vi "test write new frame.vi"() -> ()   [LabVIEW 2018, in "Data Parser.lvclass"]
uses:
  Data Parser.lvclass
  frame data.ctl
  frame title.ctl
  frame basic data.ctl
  frame o data.ctl
  frame bp data.ctl
  frame c data.ctl
  frame w data.ctl
  frame i data.ctl
  frame b data.ctl
panel:
  in  "frame data":T1
  out "new":bool
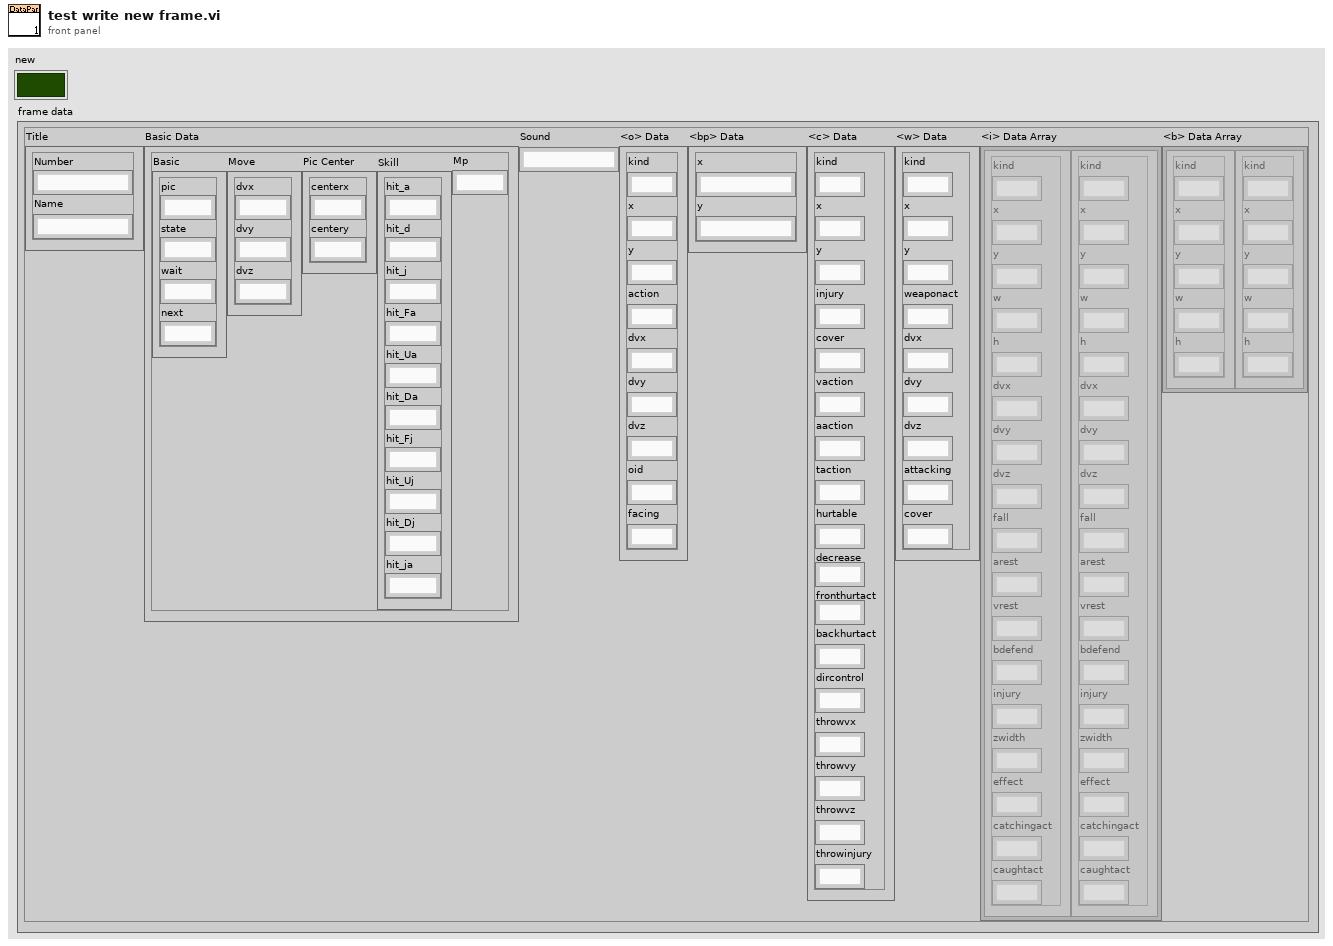
[diagram p1: front panel]
types:
  T1 = typedef "Data Parser.lvclass/frame data.ctl" = cluster{"Title":T2, "Basic Data":T3, "Sound":string, "<o> Data":T4, "<bp> Data":T5, "<c> Data":T6, "<w> Data":T7, "<i> Data Array":T8[], "<b> Data Array":T9[]}
  T2 = typedef "Data Parser.lvclass/frame title.ctl" = cluster{"Number":string, "Name":string}
  T3 = typedef "Data Parser.lvclass/frame basic data.ctl" = cluster{"Basic":cluster{"pic":string, "state":string, "wait":string, "next":string}, "Move":cluster{"dvx":string, "dvy":string, "dvz":string}, "Pic Center":cluster{"centerx":string, "centery":string}, "Skill":cluster{"hit_a":string, "hit_d":string, "hit_j":string, "hit_Fa":string, "hit_Ua":string, "hit_Da":string, "hit_Fj":string, "hit_Uj":string, "hit_Dj":string, "hit_ja":string}, "Mp":string}
  T4 = typedef "Data Parser.lvclass/frame o data.ctl" = cluster{"kind":string, "x":string, "y":string, "action":string, "dvx":string, "dvy":string, "dvz":string, "oid":string, "facing":string}
  T5 = typedef "Data Parser.lvclass/frame bp data.ctl" = cluster{"x":string, "y":string}
  T6 = typedef "Data Parser.lvclass/frame c data.ctl" = cluster{"kind":string, "x":string, "y":string, "injury":string, "cover":string, "vaction":string, "aaction":string, "taction":string, "hurtable":string, "decrease":string, "fronthurtact":string, "backhurtact":string, "dircontrol":string, "throwvx":string, "throwvy":string, "throwvz":string, "throwinjury":string}
  T7 = typedef "Data Parser.lvclass/frame w data.ctl" = cluster{"kind":string, "x":string, "y":string, "weaponact":string, "dvx":string, "dvy":string, "dvz":string, "attacking":string, "cover":string}
  T8 = typedef "Data Parser.lvclass/frame i data.ctl" = cluster{"kind":string, "x":string, "y":string, "w":string, "h":string, "dvx":string, "dvy":string, "dvz":string, "fall":string, "arest":string, "vrest":string, "bdefend":string, "injury":string, "zwidth":string, "effect":string, "catchingact":string, "caughtact":string}
  T9 = typedef "Data Parser.lvclass/frame b data.ctl" = cluster{"kind":string, "x":string, "y":string, "w":string, "h":string}
  T10 = enum16{"open", "replace", "create", "open or create", "replace or create", "replace or create with confirmation"}
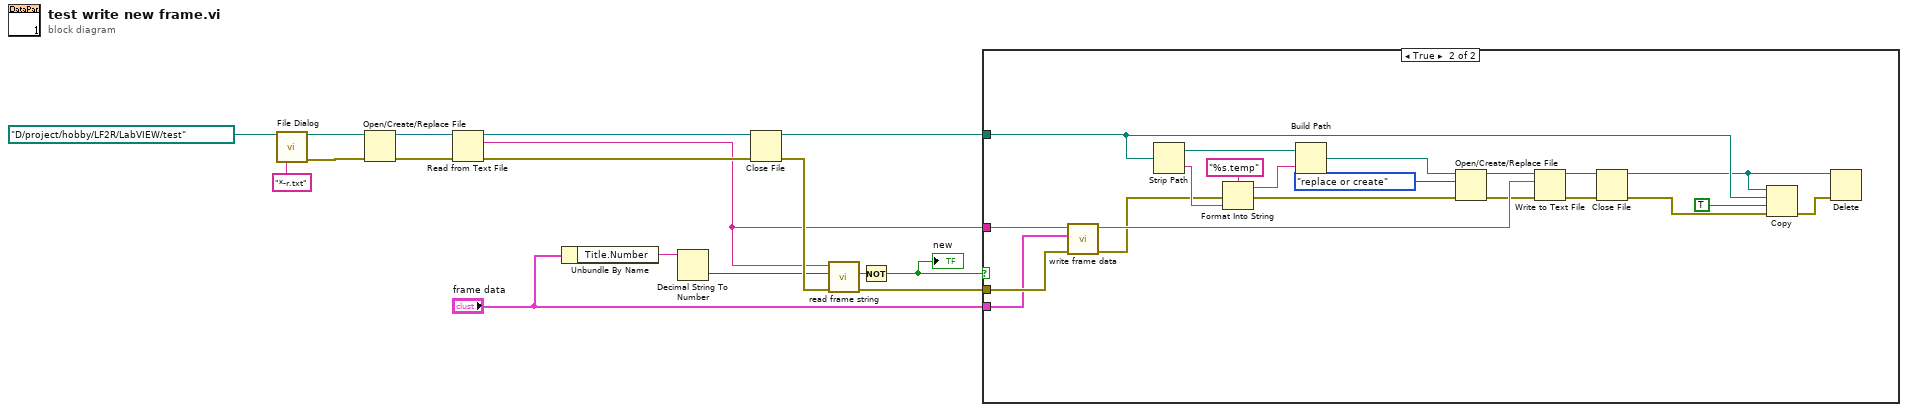
[diagram p0: block diagram]
diagram:
  n1 = call "File Dialog"("start path"=path "D:/project/hobby/LF2R/LabVIEW/test", "pattern (all files)"="*-r.txt") -> ("selected path"=w15:path, "error out"=w14:errorcluster)  [unwired: 10 in, 2 out]
  n2 = Open/Create/Replace File(file path (use dialog)=w15, error in=w14) -> (refnum out=w17:refnum<file>, error out=w16:errorcluster)  [unwired: 4 in, 1 out]
  n3 = Read from Text File(file (use dialog)=w17, error in=w16) -> (refnum out=w11:refnum<file>, text=w7:string, error out=w10:errorcluster)  [unwired: 2 in, 1 out]
  n4 = Unbundle By Name("frame data") -> ("Title.Number"=w2:string)
  n5 = Decimal String To Number(string=w2) -> (number=w1:i32)  [unwired: 2 in, 1 out]
  n6 = Close File(refnum=w11, error in=w10) -> (path=w8:path, error out=w9:errorcluster)
  n7 = call "read frame string.vi"("error in"=w9, "frame number"=w1, "file string"=w7) -> ("error out"=w4:errorcluster, "found"=w6:bool)  [unwired: 5 in, 2 out]
  n8 = Not(x=w6) -> (.not. x?=w5:bool)
  "new" <- w5
  n9 = case shown="True" w5 {
    tunnel: w8 -> [_ w38]
    tunnel: w7 -> [_ w37]
    tunnel: "frame data" -> [_ w18]
    tunnel: w4 -> [_ w19]
    frame False {
    }
    frame True {
      n10 = call "write frame data.vi"("error in"=w19, "frame data"=w18, "file string in"=w37) -> ("error out"=w20:errorcluster, "file string out"=w36:string)  [unwired: 7 in]
      n11 = Strip Path(path=w38) -> (stripped path=w31:path, name=w30:string)
      n12 = Format Into String(format string="%s.temp", error in=w20, w30) -> (resulting string=w28:string, error out=w26:errorcluster)  [unwired: 1 in]
      n13 = Build Path(base path=w31, name or relative path=w28) -> (appended path=w27:path)
      n14 = Open/Create/Replace File(file path (use dialog)=w27, error in=w26, operation (0:open)=T10."replace or create") -> (refnum out=w35:refnum<file>, error out=w34:errorcluster)  [unwired: 3 in, 1 out]
      n15 = Write to Text File(file (use dialog)=w35, text=w36, error in=w34) -> (refnum out=w33:refnum<file>, error out=w32:errorcluster)  [unwired: 1 in, 1 out]
      n16 = Close File(refnum=w33, error in=w32) -> (path=w21:path, error out=w25:errorcluster)
      n17 = Copy(8:w25, 9:TRUE ("overwrite (F)"), 10:w38, 11:w21) -> (0:w23:errorcluster)  [unwired: 1 in, 2 out]
      n18 = Delete(path (use dialog)=w21, error in=w23) -> ()  [unwired: 3 in, 3 out]
    }
  }
